vi "Sharp.vi"() -> (0 "Slide 2":dbl(slide) scale=0.0..10.0)   [LabVIEW 2014]
panel:
  out "Slide":dbl(slide) scale=0.0..10.0
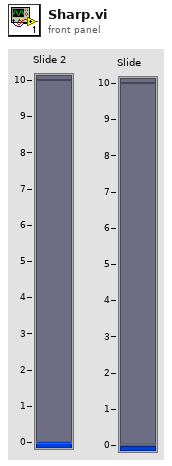
[diagram p1: front panel]
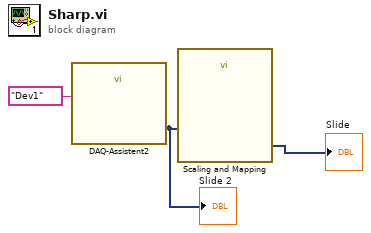
[diagram p0: block diagram]
diagram:
  n1 = call "DAQ-Assistent2"("device name"=tag "Dev1") -> ("data"=w3:dynamicdata)  [unwired: 16 in, 2 out]
  "Slide 2" <- w3
  n2 = call "Scaling and Mapping"("Signals"=w3) -> ("Scaled Signals"=→"Slide":dynamicdata)  [unwired: 9 in, 1 out]
